vi "Area.vi"(8 "error in":errorcluster, 11 "Circle in":refnum<class "Circle.lvclass">) -> (0 "error out":errorcluster, 2 "area":dbl, 3 "Circle out":refnum<class "Circle.lvclass">)   [LabVIEW 2015, in "Circle.lvclass"]
uses:
  Circle.lvclass
  Circle.lvclass/Circle.ctl
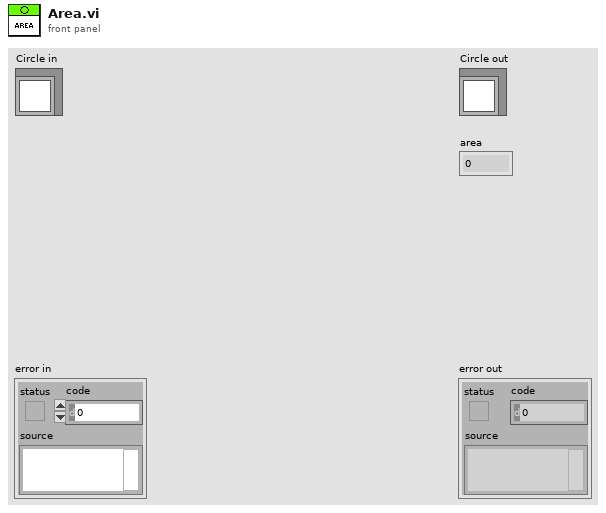
[diagram p1: front panel]
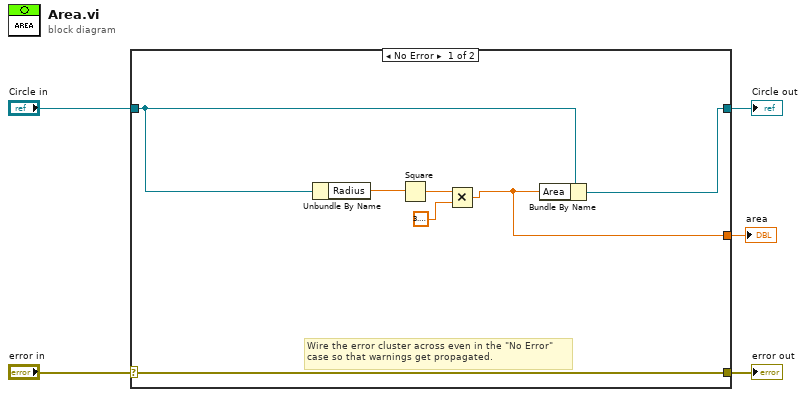
[diagram p0: block diagram]
diagram:
  n1 = case shown="No Error" "error in" {
    selector: "error in" -> [w12 w14]
    tunnel: [w12 w14] -> w4
    tunnel: [w7 w13] -> w2
    tunnel: "Circle in" -> [w8 w13]
    tunnel: [w6 _] -> w1
    frame No Error {
      # "Wire the error cluster across even in the \"No Error\"\ncase so that warnings get propagated."
      n2 = Unbundle By Name(w8) -> ("Radius"=w11:dbl)
      n3 = Square(x=w11) -> (x^2=w10:dbl)
      n4 = Multiply(x=w10, y=3.141592653589793) -> (x*y=w6:dbl)
      n5 = Bundle By Name(cluster=w8, "Area"=w6) -> (w7:refnum<class "Circle.lvclass">)
    }
    frame Error {
    }
  }
  "error out" <- w4
  "Circle out" <- w2
  "area" <- w1
